vi "PID control-backup.vi"() -> ()   [LabVIEW 2017]
uses:
  <vilib>/Simulation/Scripting/Companion Diagram/SimConfigNode/SimParams.ctl
  <vilib>/Simulation/Scripting/Companion Diagram/SimConfigNode/_simSolvers.ctl
  <vilib>/Simulation/Implementation/Shared/SIMSCR Execution Mode.ctl
  <vilib>/Simulation/Param Hierarchy/Typedefs/SIMPH Param Control Actions.ctl
  <vilib>/Simulation/Implementation/Shared/NILVSim_ParamChanged.vi
  <vilib>/Simulation/Implementation/Shared/NILVSIM_BeginStep.vi
  <vilib>/Simulation/Implementation/Shared/NILVSim_Manager.vi
  <vilib>/Utility/error.llb/Clear Errors.vi
  <vilib>/Simulation/Implementation/Shared/NILVSim_FinalizeModel.vi
  <vilib>/DAQmx/read.llb/DAQmx Read (Counter DBL 1Chan 1Samp).vi
  <vilib>/DAQmx/read.llb/DAQmx Read (Digital Bool 1Line 1Point).vi
  917b7e52-755f-4d44-bea8-9e7c9beac24e.vi
  a58f9967-76f1-4ebc-ad3d-26e75a3ca160.vi
  <vilib>/DAQmx/write.llb/DAQmx Write (Analog DBL 1Chan 1Samp).vi
  <vilib>/DAQmx/create/channels.llb/DAQmx Create Channel (AO-Voltage-Basic).vi
  <vilib>/DAQmx/create/channels.llb/DAQmx Create Channel (DI-Digital Input).vi
  <vilib>/DAQmx/create/channels.llb/DAQmx Create Channel (CI-Count Edges).vi
  <vilib>/Simulation/Implementation/Shared/SIM Unbundle Sim Info.vi
  <vilib>/Simulation/Implementation/Shared/NILVSim_Initialize.vi
  <vilib>/Simulation/Utility/Implementation/NILVSim Get Time and IsAcceptedStep.vi
  <vilib>/Simulation/Implementation/Shared/SIMSH Read Queue.vi
  <vilib>/Simulation/Implementation/Shared/NILVSim_GetModelError.vi
  <vilib>/Simulation/Implementation/Shared/SIM Bundle Sim Info.vi
  <vilib>/DAQmx/miscellaneous.llb/DAQmx Fill In Error Info.vi
  <vilib>/Simulation/Implementation/XNodeFramework/SimXNode/SimX.xnode
  <vilib>/Simulation/Model Libraries/PID/SIM PID (Parallel).vi
  <vilib>/Simulation/Model Libraries/PID/SIM PID.vi
  <vilib>/Simulation/Scripting/Companion Diagram/SimConfigNode/SimDog.xnode
  <vilib>/Simulation/Model Libraries/PID/SIM PID (Academic).vi
  <vilib>/Simulation/Implementation/Shared/NI_SIM_Implementation.lvlib
panel:
  out "down":bool
  out "right":bool
  out "x entered":dbl
  out "y enetred":dbl
  out "Numeric 2":i32
  out "greater -1 x":bool
  out "less 1 x":bool
  out "d":bool
  out "c":bool
  out "b":bool
  out "direction selected":dbl
  out "circle reset":bool
  in  "part circle":T1(ring)=enum."a"
  in  "Raduis":dbl
  out "at 2f":bool
  out "Step 2J":bool
  out "Step 2H":bool
  out "Shape drawing steps":enum16{"corner", "1st switch", "reverse"}(ring)
  out "Step 2D":bool
  out "Step 2C":bool
  out "c":bool
  in  "height":dbl
  in  "length":dbl
  in  "part":T2(ring)=enum."a"
  out "Step 2A":bool
  out "Step 2B":bool
  in  "Has encoders been reset?":enum16{"don't reset", "reset"}(ring)
  out "x distance currently being travelled":dbl
  out "y distance currently being travelled":dbl
  out "error calced":dbl
  out "p1 dis 2":dbl
  out "p1 dis":dbl
  out "error y":dbl
  out "calc distance y":dbl
  out "calc distanc x":dbl
  out "error x":dbl
  out "reached y":bool
  out "reached x":bool
  out "Numeric":dbl
  in  "Draw rectangle":bool
  in  "Draw circle":bool
  out "In drawing mode":bool
  in  "Right-Down":bool
  in  "Left-Up":bool
  in  "Left-Down":bool
  in  "Right-Up":bool
  in  "right":bool
  in  "left":bool
  in  "motor 2":dbl(slide)=1.5 scale=-10.0..10.0
  in  "down":bool
  in  "up":bool
  in  "Y Length":dbl=30.0
  in  "X Length":dbl=30.0
  in  "Motor 2 encoder":tag="Dev1/ctr1"
  out "Pulses M2":dbl format="%.2f"
  in  "Motor 1 encoder":tag="Dev1/ctr0"
  out "Pulses M1":dbl format="%.2f"
  out "Right":bool
  out "Bottom":bool
  out "Left":bool
  out "Top":bool
  in  "Switch 4/Line 3":tag="Dev1/port0/line3"
  in  "Switch 3/Line 2":tag="Dev1/port0/line2"
  in  "Switch 2/Line 1":tag="Dev1/port0/line1"
  in  "Switch 1/Line 0":tag="Dev1/port0/line0"
  in  "Motor stop":bool
  in  "Motor 1":tag="Dev1/ao0"
  in  "max Voltage":dbl=10.0
  in  "Min Voltage":dbl=-10.0
  in  "Motor 2":tag="Dev1/ao1"
  in  "motor 1":dbl(slide)=1.5 scale=-10.0..10.0
  in  "stop":bool
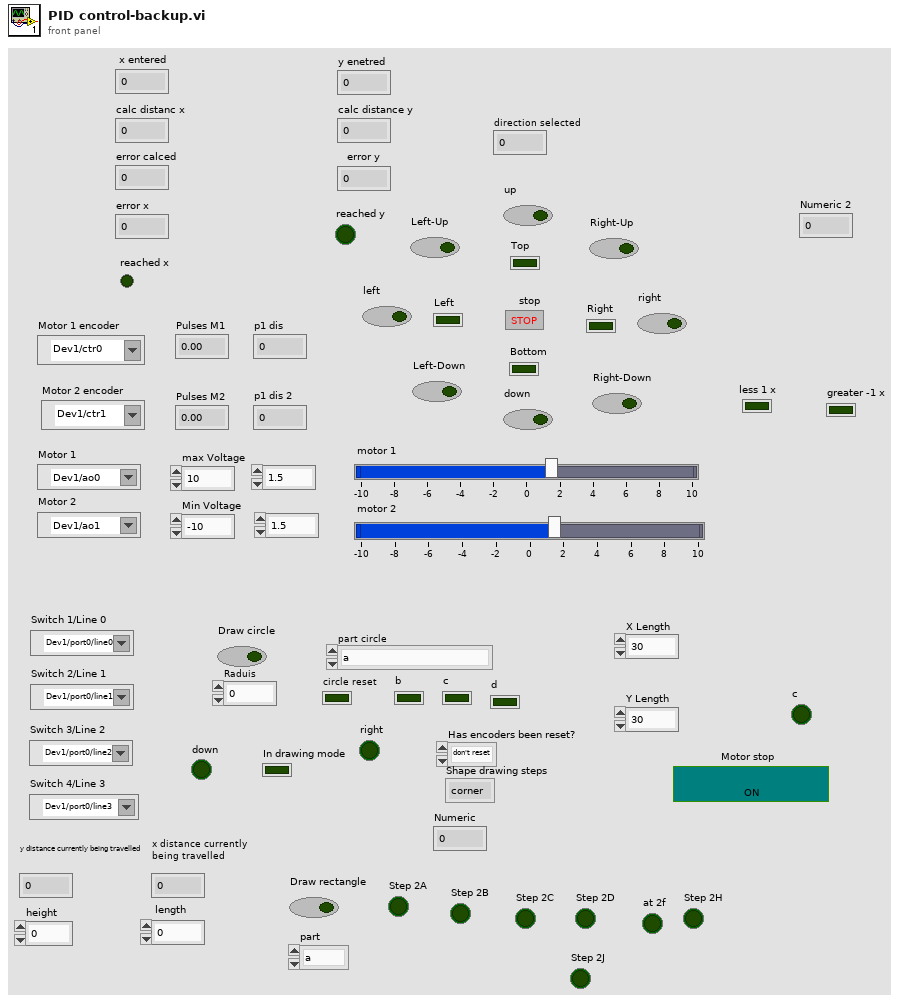
[diagram p1: front panel]
types:
  T1 = enum16{"d", "c", "b", "going right", "going down", "a"}
  T2 = enum16{"nothing", "j", "i", "h", "g", "f", "e", "d", "c", "b", "a"}
  T3 = enum16{"Simulate to Completion", "Single Time-Step Simulation (Fixed Step Only)"}
  T4 = typedef "SIMSCR Execution Mode.ctl" = enum16{"Simulate to Completion", "Single Time-Step Simulation (Fixed Step Only)"}
  T5 = typedef "SIMPH Param Control Actions.ctl" = enum16{"get params", "set params"}
  T6 = cluster{"SIMSH Sim Time":dbl, "SIM PID Derivative Gain.vi":cluster{"output":dbl}, "SIM PID Derivative Gain.vi - SIMSH":cluster{"SIMSH Sim Time":dbl, "t 3":dbl, "Select 2":cluster{"s? t:f":dbl}, "Equal?":cluster{"x = y?":bool}, "Or":cluster{"x .or. y?":bool}, "Equal To 0?":cluster{"x = 0?":bool}}, "High Frequency [s] (Tf)":dbl, "Gain":cluster{"output":dbl}, "Summation":cluster{"Result":dbl}, "Integral Gain - series.vi":cluster{"output":dbl}, "Integral Gain - series.vi - SIMSH":cluster{"SIMSH Sim Time":dbl, "Select 2":cluster{"s? t:f":dbl}, "integral in gain?":bool, "Integrator":cluster{"output y(t)":dbl}, "Gain 2":cluster{"output":dbl}, "Select":cluster{"s? t:f":dbl}, "Equal To 0?":cluster{"x = 0?":bool}, "Reciprocal":cluster{"1/x":dbl}}}
  T7 = typedef "SimParams.ctl" = cluster{"Initial Time (s)":dbl, "Final Time (s)":dbl, "Step Size (s)":dbl, "ODE Solver":T8, "Minimum Step Size (s)":dbl, "Maximum Step Size (s)":dbl, "Relative Tolerance":dbl, "Absolute Tolerance":dbl, "Software Timing":bool, "Initial Step Size (s)":dbl, "Automatic Fixed Step Size?":bool, "Automatic Discrete Step Size?":bool, "Discrete Step Size (s)":dbl, "Calculate using Time Step":bool, "Solver Wired?":bool, "Prev.Frm.Expected End":u64, "Prev.Frm.Actual End":u64, "Prev.Frm.Finished Late?":bool, "Prev.Iter.Expected End":u64, "Prev.Iter.Actual End":u64, "Prev.Iter.Finished Late?":bool, "Expected Iteration Start":u64, "Actual Iteration Start":u64, "Expected Frame Start":u64, "Actual Frame Start":u64, "Source Name":string, "Name":string, "Period":i64, "Deadline":i64, "Offset":i64, "Start":i64, "Priority":i32, "Timeout":i32, "Processor":i32, "Mode":enum32{"No Change", "Process missed periods, maintain original phase", "Discard missed periods, maintain original phase", "Process missed periods, ignore original phase", "Discard missed periods, ignore original phase"}, "Wakeup reason":enum32{"Normal", "Aborted", "Asynchronous wakeup", "Timing source error", "Timed loop error", "Timeout"}, "Error":errorcluster, "Source Type":string, "Secondary Source Type":string, "Global End Time":u64, "Global Start Time":u64, "Full Solver Reset":bool, "Execution Mode":T4, "Nan/Inf Check":bool, "Custom Solver Library":string, "Solver Is Variable":bool, "custom solver name":string, "Signal Collection Decimation":u32}
  T8 = typedef "_simSolvers.ctl" = enum16{"Runge-Kutta 1 (Euler)", "Runge-Kutta 2", "Runge-Kutta 3", "Runge-Kutta 4", "Runge-Kutta 23 (variable)", "Runge-Kutta 45 (variable)", "BDF (variable)", "Adams-Moulton (variable)", "Rosenbrock (variable)", "Discrete States Only", "SDIRK 4 (variable)", "Radau 5 (variable)", "Radau 9 (variable)", "Radau 13 (variable)", "Radau [Variable Order] (variable)", "Gear's Method (variable)", "Linearizer", "State Query", "Trim Eval", "Custom Solver"}
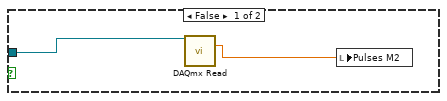
[diagram p2: hidden frame]
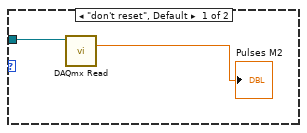
[diagram p3: hidden frame]
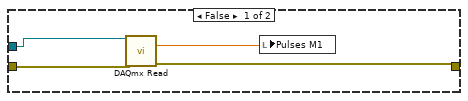
[diagram p4: hidden frame]
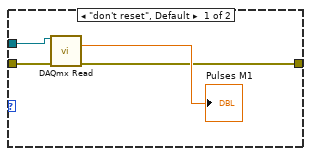
[diagram p5: hidden frame]
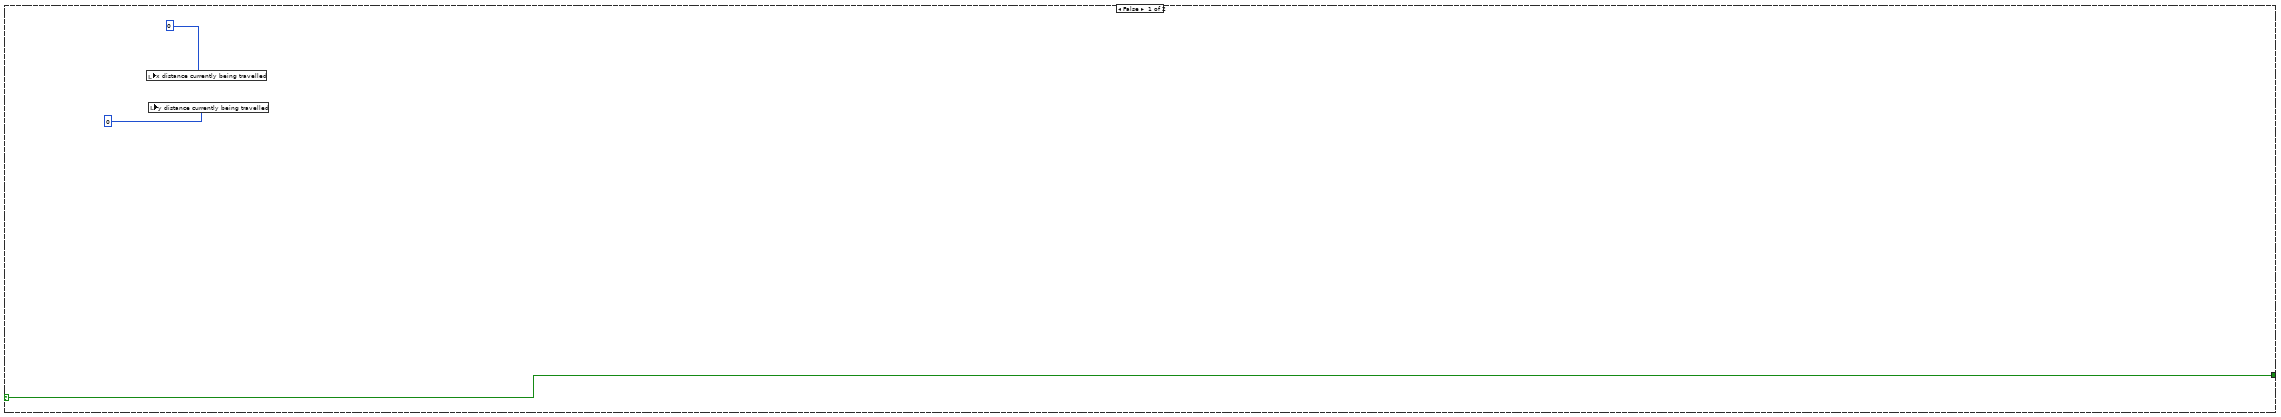
[diagram p6: hidden frame]
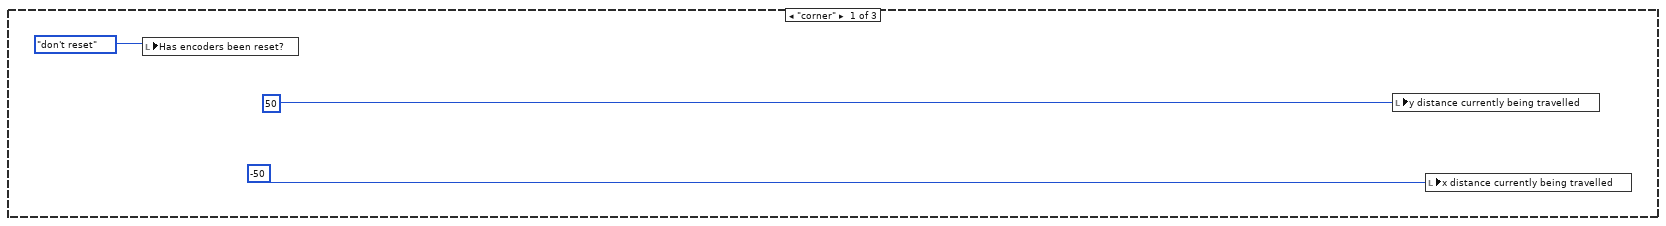
[diagram p7: hidden frame]
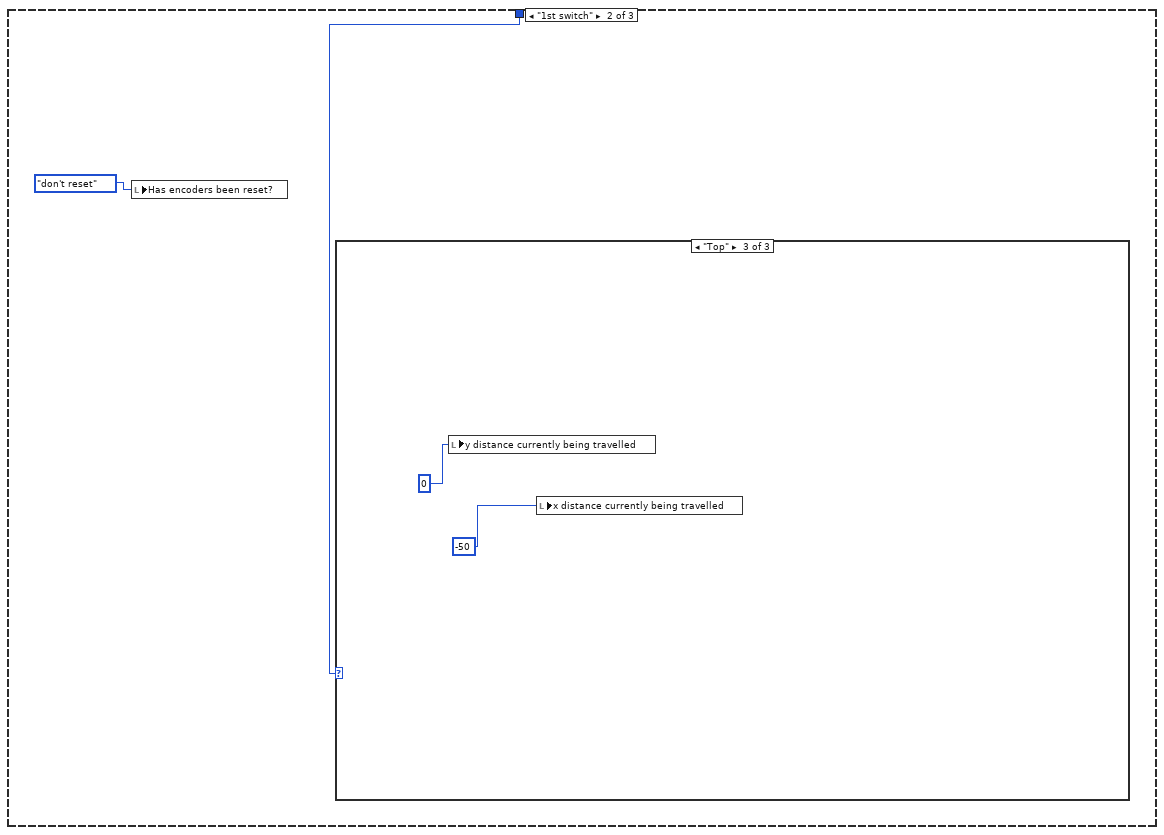
[diagram p8: hidden frame]
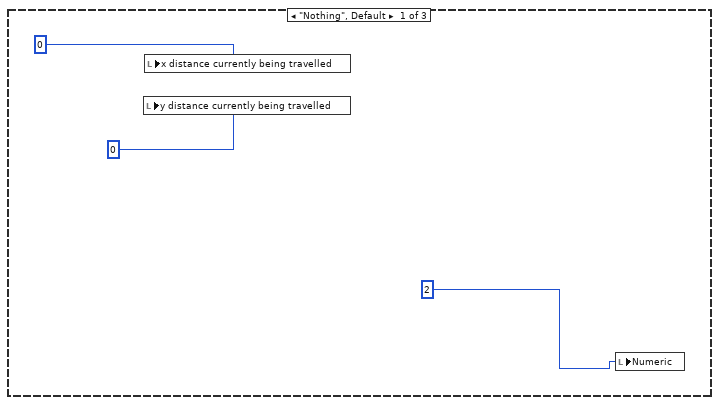
[diagram p9: hidden frame]
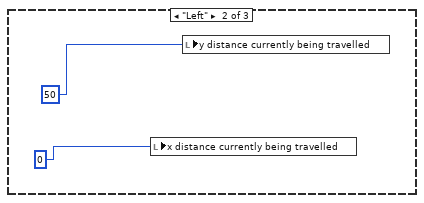
[diagram p10: hidden frame]
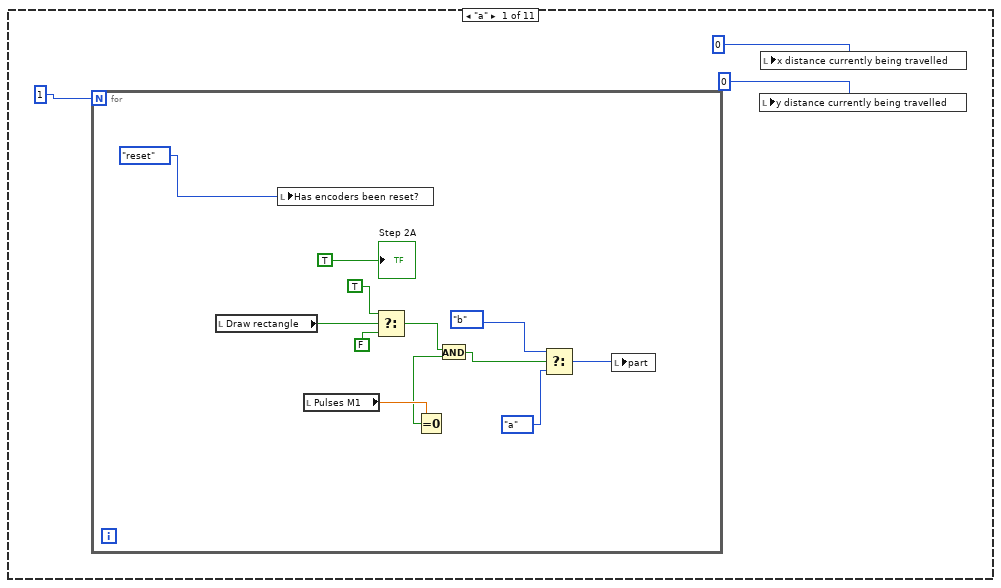
[diagram p11: hidden frame]
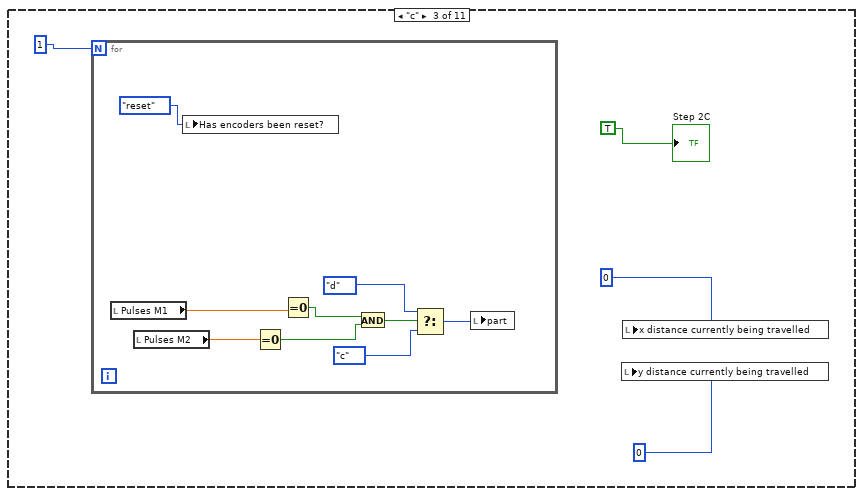
[diagram p12: hidden frame]
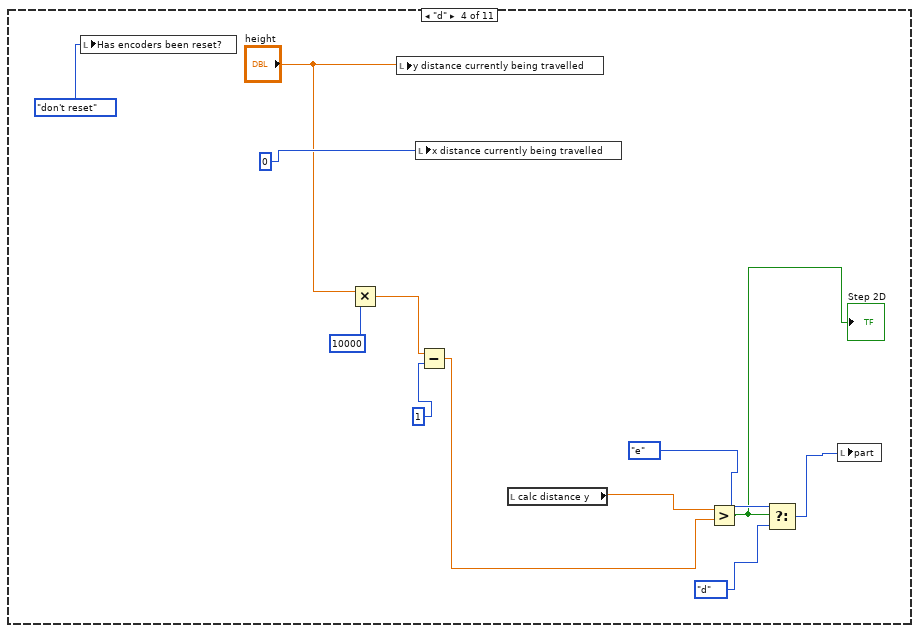
[diagram p13: hidden frame]
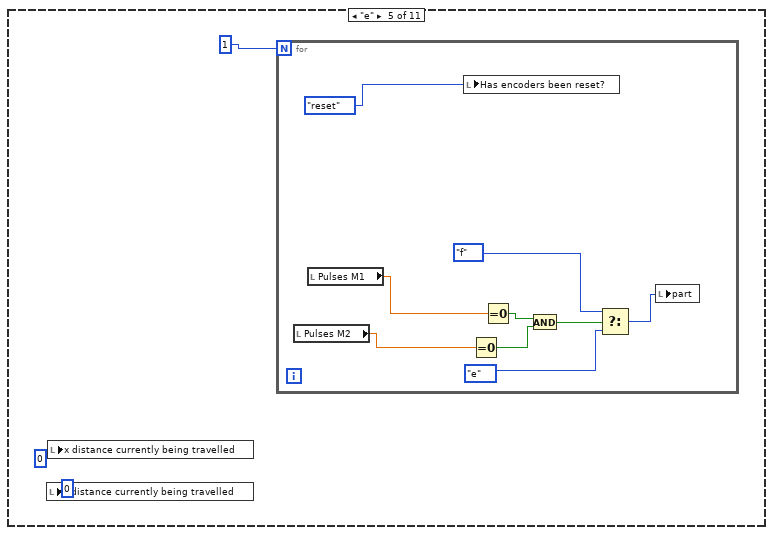
[diagram p14: hidden frame]
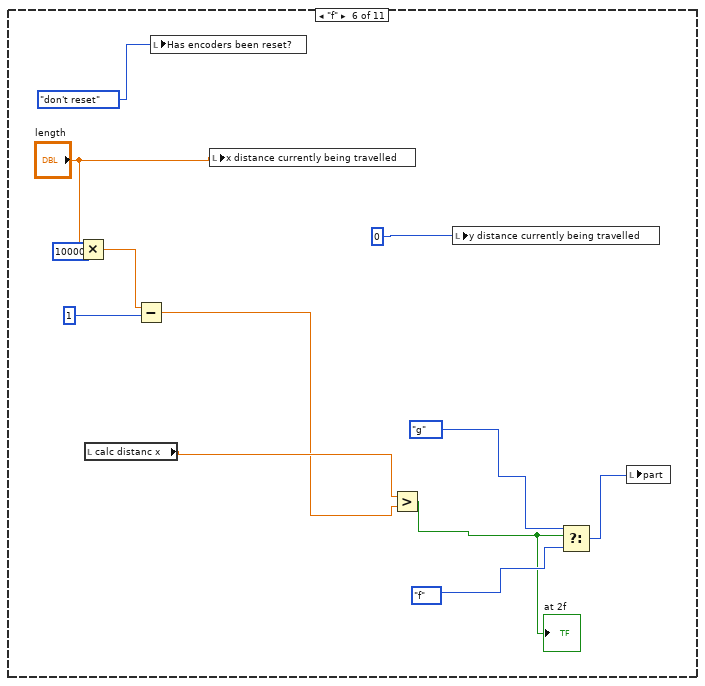
[diagram p15: hidden frame]
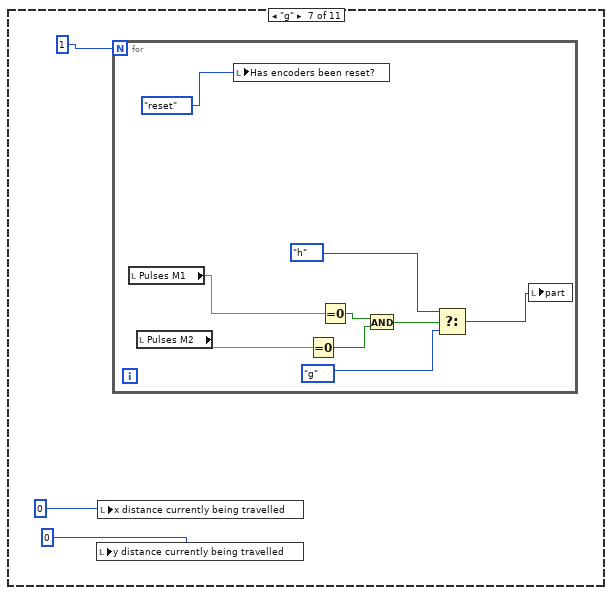
[diagram p16: hidden frame]
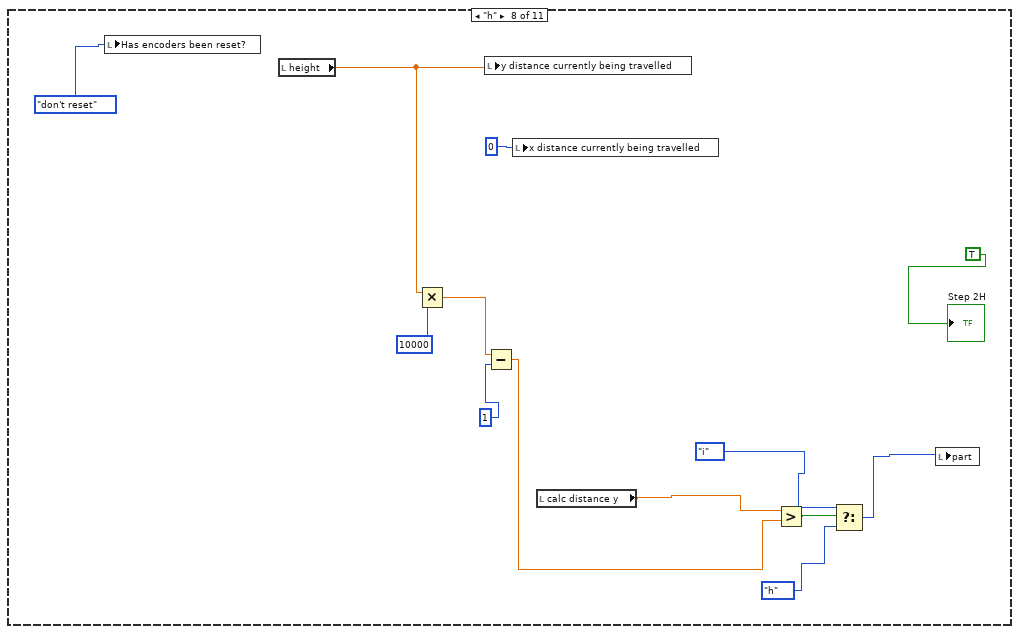
[diagram p17: hidden frame]
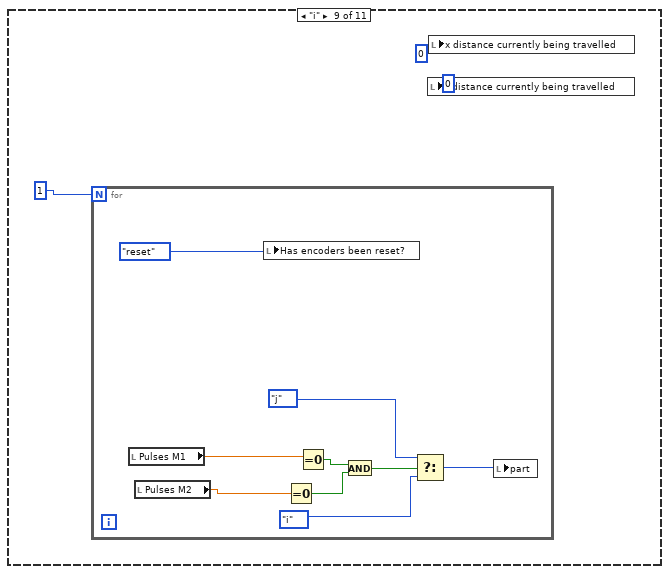
[diagram p18: hidden frame]
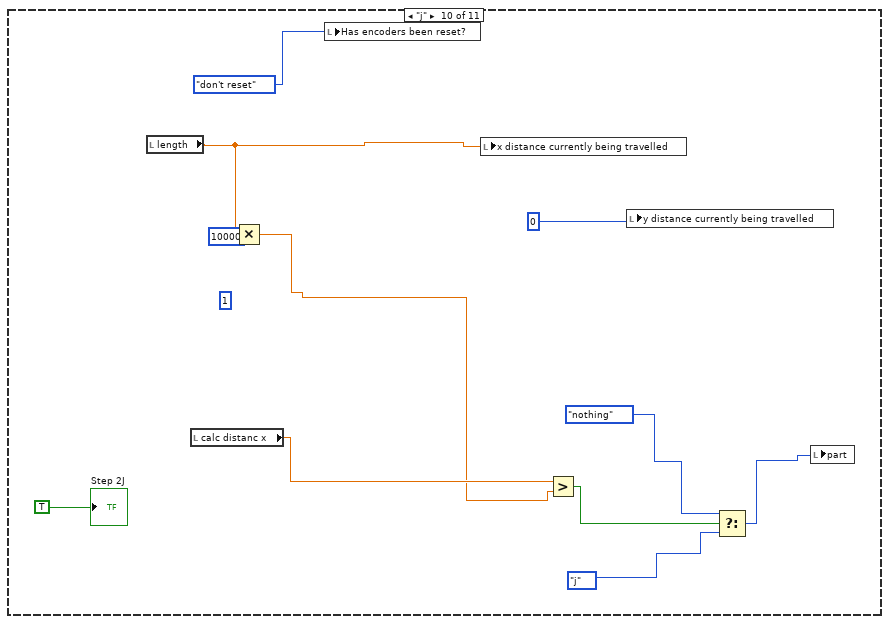
[diagram p19: hidden frame]
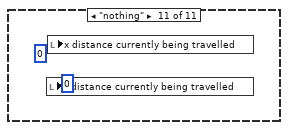
[diagram p20: hidden frame]
diagram:
  n1 = call-poly <vilib>:"DAQmx Create Virtual Channel.vi"("lines"="Switch 1/Line 0") -> ("task out"=w36:refnum<k21>, "error out"=w32:errorcluster)  [unwired: 13 in]
  n2 = call-poly <vilib>:"DAQmx Create Virtual Channel.vi"("lines"="Switch 2/Line 1") -> ("task out"=w35:refnum<k21>, "error out"=w31:errorcluster)  [unwired: 13 in]
  n3 = call-poly <vilib>:"DAQmx Create Virtual Channel.vi"("lines"="Switch 3/Line 2") -> ("task out"=w34:refnum<k21>, "error out"=w30:errorcluster)  [unwired: 13 in]
  n4 = call-poly <vilib>:"DAQmx Create Virtual Channel.vi"("lines"="Switch 4/Line 3") -> ("task out"=w33:refnum<k21>, "error out"=w29:errorcluster)  [unwired: 13 in]
  n5 = call <vilib>:"DAQmx Start Task.vi"("task/channels in"=w36, "error in"=w32) -> ("task out"=w28:refnum<k21>, "error out"=w26:errorcluster)  [unwired: 12 in]
  n6 = call <vilib>:"DAQmx Start Task.vi"("task/channels in"=w35, "error in"=w31) -> ("task out"=w24:refnum<k21>, "error out"=w21:errorcluster)  [unwired: 12 in]
  n7 = call <vilib>:"DAQmx Start Task.vi"("task/channels in"=w34, "error in"=w30) -> ("task out"=w23:refnum<k21>, "error out"=w20:errorcluster)  [unwired: 12 in]
  n8 = call <vilib>:"DAQmx Start Task.vi"("task/channels in"=w33, "error in"=w29) -> ("task out"=w22:refnum<k21>, "error out"=w19:errorcluster)  [unwired: 12 in]
  n9 = call-poly <vilib>:"DAQmx Create Virtual Channel.vi"("maximum value"="max Voltage", "minimum value"="Min Voltage", "physical channels"="Motor 1") -> ("task out"=w46:refnum<k21>, "error out"=w42:errorcluster)  [unwired: 11 in]
  n10 = call-poly <vilib>:"DAQmx Create Virtual Channel.vi"("counter"="Motor 2 encoder") -> ("task out"=w6:refnum<k21>)  [unwired: 13 in, 1 out]
  n11 = call-poly <vilib>:"DAQmx Create Virtual Channel.vi"("maximum value"="max Voltage", "minimum value"="Min Voltage", "physical channels"="Motor 2") -> ("task out"=w49:refnum<k21>, "error out"=w41:errorcluster)  [unwired: 11 in]
  n12 = call-poly <vilib>:"DAQmx Create Virtual Channel.vi"("counter"="Motor 1 encoder") -> ("task out"=w7:refnum<k21>, "error out"=w2:errorcluster)  [unwired: 13 in]
  n13 = call <vilib>:"DAQmx Start Task.vi"("task/channels in"=w6) -> ("task out"=w1:refnum<k21>)  [unwired: 13 in, 1 out]
  n14 = call <vilib>:"DAQmx Start Task.vi"("task/channels in"=w7) -> ("task out"=w3:refnum<k21>)  [unwired: 13 in, 1 out]
  n15 = while {
    tunnel: w49 -> [w239]
    tunnel: [w236] -> w48
    tunnel: w46 -> [w233]
    tunnel: [w232] -> w45
    tunnel: w42 -> [w230]
    tunnel: w41 -> [w229]
    tunnel: w28 -> [w223]
    tunnel: [w222] -> w27
    tunnel: w26 -> [w221]
    tunnel: [w220] -> w25
    tunnel: w24 -> [w219]
    tunnel: w23 -> [w218]
    tunnel: w22 -> [w217]
    tunnel: w21 -> [w216]
    tunnel: w20 -> [w215]
    tunnel: w19 -> [w214]
    tunnel: [w213] -> w18
    tunnel: [w212] -> w17
    tunnel: [w211] -> w16
    tunnel: [w210] -> w15
    tunnel: [w209] -> w14
    tunnel: [w208] -> w13
    tunnel: [w131] -> w10
    tunnel: w3 -> [w133]
    tunnel: w2 -> [w132]
    tunnel: w1 -> [w129]
    stop <- "stop" stop-if-true
    n16 = Or(x="Draw circle", y="Draw rectangle") -> (x .or. y?=w152:bool)
    n17 = local read "error y"() -> (w99:dbl)
    n18 = local read "error y"() -> (w98:dbl)
    n19 = local read "error x"() -> (w100:dbl)
    n20 = local read "error y"() -> (w114:dbl)
    n21 = local read "error y"() -> (w111:dbl)
    n22 = local read "error x"() -> (w107:dbl)
    n23 = local read "error x"() -> (w106:dbl)
    n24 = local read "error y"() -> (w115:dbl)
    n25 = local read "error x"() -> (w116:dbl)
    n26 = Less Than 0?(x=w99) -> (x < 0?=w97:bool)
    n27 = Less Than 0?(x=w100) -> (x < 0?=w96:bool)
    n28 = Greater Than 0?(x=w98) -> (x > 0?=w95:bool)
    n29 = Less Than 0?(x=w111) -> (x < 0?=w109:bool)
    n30 = Equal To 0?(x=w116) -> (x = 0?=w110:bool)
    n31 = Greater Than 0?(x=w114) -> (x > 0?=w113:bool)
    n32 = local read "error y"() -> (w92:dbl)
    n33 = local read "error x"() -> (w91:dbl)
    n34 = Greater Than 0?(x=w107) -> (x > 0?=w105:bool)
    n35 = Equal To 0?(x=w115) -> (x = 0?=w104:bool)
    n36 = Less Than 0?(x=w106) -> (x < 0?=w103:bool)
    n37 = And(x=w97, y=w96) -> (x .and. y?=w93:bool)
    n38 = And(x=w96, y=w95) -> (x .and. y?=w94:bool)
    n39 = And(x=w113, y=w110) -> (x .and. y?=w112:bool)
    n40 = And(x=w110, y=w109) -> (x .and. y?=w108:bool)
    n41 = local read "error y"() -> (w87:dbl)
    n42 = And(x=w105, y=w104) -> (x .and. y?=w102:bool)
    n43 = And(x=w104, y=w103) -> (x .and. y?=w101:bool)
    n44 = Greater Than 0?(x=w92) -> (x > 0?=w90:bool)
    n45 = Greater Than 0?(x=w91) -> (x > 0?=w88:bool)
    n46 = Less Than 0?(x=w87) -> (x < 0?=w86:bool)
    n47 = And(x=w90, y=w88) -> (x .and. y?=w89:bool)
    n48 = And(x=w88, y=w86) -> (x .and. y?=w85:bool)
    n49 = Select(t=1, s=w112, f=0) -> (s? t:f=w192:i32)
    n50 = Select(t=10, s=w101, f=0) -> (s? t:f=w190:i32)
    n51 = Select(t=2, s=w108, f=0) -> (s? t:f=w191:i32)
    n52 = Select(t=100, s=w89, f=0) -> (s? t:f=w188:i32)
    n53 = Select(t=200, s=w93, f=0) -> (s? t:f=w187:i32)
    n54 = Select(t=20, s=w102, f=0) -> (s? t:f=w189:i32)
    n55 = Select(t=1000, s=w94, f=0) -> (s? t:f=w186:i32)
    n56 = Select(t=2000, s=w85, f=0) -> (s? t:f=w172:i32)
    n57 = Add(x=w192, y=w191) -> (x+y=w185:i32)
    n58 = Add(x=w190, y=w189) -> (x+y=w184:i32)
    n59 = Add(x=w188, y=w187) -> (x+y=w183:i32)
    n60 = Add(x=w186, y=w172) -> (x+y=w171:i32)
    n61 = Add(x=w185, y=w184) -> (x+y=w182:i32)
    n62 = local read "y distance currently being travelled"() -> (w135:dbl)
    n63 = Add(x=w183, y=w171) -> (x+y=w170:i32)
    n64 = local read "Draw rectangle"() -> (w143:bool)
    n65 = local read "Draw circle"() -> (w144:bool)
    n66 = call-poly <vilib>:"DAQmx Read.vi"("task/channels in"=w223, "error in"=w221) -> ("task out"=w222:refnum<k21>, "data"=w154:bool, "error out"=w220:errorcluster)  [unwired: 11 in]
    "Top" <- w154
    n67 = call-poly <vilib>:"DAQmx Read.vi"("task/channels in"=w219, "error in"=w216) -> ("task out"=w213:refnum<k21>, "data"=w163:bool, "error out"=w210:errorcluster)  [unwired: 11 in]
    "Bottom" <- w163
    n68 = call-poly <vilib>:"DAQmx Read.vi"("task/channels in"=w218, "error in"=w215) -> ("task out"=w212:refnum<k21>, "data"=w162:bool, "error out"=w209:errorcluster)  [unwired: 11 in]
    "Right" <- w162
    n69 = call-poly <vilib>:"DAQmx Read.vi"("task/channels in"=w217, "error in"=w214) -> ("task out"=w211:refnum<k21>, "data"=w161:bool, "error out"=w208:errorcluster)  [unwired: 11 in]
    "Left" <- w161
    n70 = Add(x=w182, y=w170) -> (x+y=w84:i32)
    "direction selected" <- w84
    n71 = Or(x=w144, y=w143) -> (x .or. y?=w142:bool)
    n72 = Select(t=w135, s=w142, f="Y Length") -> (s? t:f=w140:dbl)
    n73 = Multiply(x=w140, y=10) -> (x*y=w54:dbl)
    "y enetred" <- w54
    n74 = local read "Pulses M1"() -> (w130:dbl)
    n75 = local read "Pulses M2"() -> (w145:dbl)
    n76 = Divide(x=w130, y=52.56) -> (x/y=→"p1 dis":dbl)
    n77 = feedback #1() -> (w58:dbl)  [unwired: 1 in]
    "calc distance y" <- w58
    n78 = formula code="if (Ylength==0)\nYerror=0;\n else  \nif(Ylength<0)\nYerror= Ylength+calculating_y_dis;\nelse\nYerror= Ylength-calculating_y_dis;\n\nif (calculating_y_dis>1000)\nstay=0;\nif (stay==0 )\nYerror=0;"("Ylength"=w54, "calculating_y_dis"=w58, "stay"=1) -> ("Yerror"=w118:dbl)
    n79 = Divide(x=w145, y=52.56) -> (x/y=→"p1 dis 2":dbl)
    n80 = formula code="X=((PulseM1/52.56)+(PulseM2/52.56))/2.0;\nY=((PulseM1/52.56)+(PulseM2/52.56))/2.0;"("PulseM1"=w130, "PulseM2"=w145) -> ("X"=w63:dbl, "Y"=w67:dbl)
    n81 = local read "x distance currently being travelled"() -> (w134:dbl)
    n82 = local read "Draw rectangle"() -> (w137:bool)
    n83 = Multiply(x=1000, y=w67) -> (x*y=w70:dbl)
    n84 = local read "Draw circle"() -> (w136:bool)
    n85 = xnode "PID"("Error"=w118) -> ("Output"=w69:dbl)  [unwired: 2 in, 11 out]
    n86 = Or(x=w137, y=w136) -> (x .or. y?=w125:bool)
    n87 = Select(t=w134, s=w125, f="X Length") -> (s? t:f=w138:dbl)
    n88 = Multiply(x=w138, y=10) -> (x*y=w53:dbl)
    "x entered" <- w53
    n89 = Multiply(x=1000, y=w63) -> (x*y=w64:dbl)
    n90 = Greater?(x=1, y=w69) -> (0:w82:bool)
    n91 = Less?(x=-1, y=w69) -> (x < y?=w80:bool)
    n92 = case shown="2000" w84 {
      tunnel: "motor 1" -> [w996 w999 w1002 w1009 w1013 w1017 w1023 w1029 w1035 w1040 w1047]
      tunnel: "motor 2" -> [w993 w1001 w1004 w1007 w1012 w1015 w1021 w1027 w1033 w1041 w1046]
      tunnel: [w992 w1001 w1003 w1006 w1012 w1014 w1020 w1026 w1032 w1038 w1045] -> w51
      tunnel: [w995 w998 w1002 w1008 w1013 w1016 w1022 w1028 w1034 w1039 w1044] -> w52
      frame 0, Default {
        n93 = Multiply(x=0, y=w996) -> (x*y=w995:dbl)
        n94 = Multiply(x=0, y=w993) -> (x*y=w992:dbl)
      }
      frame 1 {
        n95 = Multiply(x=-1, y=w999) -> (x*y=w998:dbl)
      }
      frame 2 {
        n96 = Multiply(x=-1.003, y=w1004) -> (x*y=w1003:dbl)
      }
      frame 10 {
        n97 = Multiply(x=-1, y=w1009) -> (x*y=w1008:dbl)
        n98 = Multiply(x=-1.1, y=w1007) -> (x*y=w1006:dbl)
      }
      frame 20 {
      }
      frame 100 {
        n99 = Multiply(x=0, y=w1017) -> (x*y=w1016:dbl)
        n100 = Multiply(x=1, y=w1015) -> (x*y=w1014:dbl)
      }
      frame 200 {
        n101 = Multiply(x=0, y=w1023) -> (x*y=w1022:dbl)
        n102 = Multiply(x=-1, y=w1021) -> (x*y=w1020:dbl)
      }
      frame 1000 {
        n103 = Multiply(x=-1, y=w1029) -> (x*y=w1028:dbl)
        n104 = Multiply(x=0, y=w1027) -> (x*y=w1026:dbl)
      }
      frame 2000 {
        n105 = Multiply(x=1, y=w1035) -> (x*y=w1034:dbl)
        n106 = Multiply(x=0, y=w1033) -> (x*y=w1032:dbl)
      }
      frame 4000 {
        n107 = Multiply(x=-1, y=w1040) -> (x*y=w1039:dbl)
        n108 = Multiply(x=0, y=w1041) -> (x*y=w1038:dbl)
      }
      frame 8000 {
        n109 = Multiply(x=-1, y=w1047) -> (x*y=w1044:dbl)
        n110 = Multiply(x=0, y=w1046) -> (x*y=w1045:dbl)
      }
    }
    n111 = And(x=w82, y=w80) -> (x .and. y?=w68:bool)
    "reached y" <- w68
    n112 = Select(t=w70, s=w68, f=w67) -> (s? t:f=w66:dbl)
    n113 = feedback-in #1(w66) -> ()
    n114 = Multiply(x=0, y=w69) -> (x*y=w78:dbl)
    n115 = Select(t=w78, s=w68, f=w69) -> (s? t:f=→"error y":dbl)
    n116 = local read "Numeric"() -> (w122:dbl)
    n117 = Or(x=w163, y=w162) -> (x .or. y?=w206:bool)
    n118 = local read "Draw circle"() -> (w127:bool)
    n119 = local read "Draw rectangle"() -> (w126:bool)
    n120 = And(x=w161, y=w154) -> (x .and. y?=w123:bool)
    n121 = Exclusive Or(1:w154, 2:w161) -> (0:w168:bool)
    n122 = Select(t=1, s=w161, f=0) -> (s? t:f=w153:i32)
    n123 = Select(t=2, s=w154, f=w153) -> (s? t:f=w158:i32)
    n124 = Select(t=1, s=w168, f=w122) -> (s? t:f=w167:dbl)
    n125 = Select(t=2, s=w123, f=w167) -> (s? t:f=w165:dbl)
    n126 = feedback #2() -> (w61:bool)  [unwired: 1 in]
    "reached x" <- w61
    n127 = Select(t=w64, s=w61, f=w63) -> (s? t:f=w57:dbl)
    "calc distanc x" <- w57
    n128 = formula code="if (actual_xLength>1000)\nstay1=0;\nif (stay1==0)\nXerror=0;\nelse \nif(desired_xlength>0)\nXerror=desired_xlength-actual_xLength;\nelse\nXerror=desired_xlength+actual_xLength;"("actual_xLength"=w57, "desired_xlength"=w53, "stay1"=1) -> ("Xerror"=w117:dbl)
    "error calced" <- w117
    n129 = xnode "PID 2"("Error"=w117) -> ("Output"=w73:dbl)  [unwired: 2 in, 11 out]
    n130 = Greater?(x=1, y=w73) -> (0:w59:bool)
    "greater -1 x" <- w59
    n131 = Less?(x=-1, y=w73) -> (x < y?=w60:bool)
    "less 1 x" <- w60
    n132 = And(x=w59, y=w60) -> (x .and. y?=w62:bool)
    n133 = Multiply(x=0, y=w73) -> (x*y=w75:dbl)
    n134 = feedback-in #2(w62) -> ()
    n135 = Or(x=w127, y=w126) -> (x .or. y?=w128:bool)
    n136 = Select(t=w75, s=w61, f=w73) -> (s? t:f=→"error x":dbl)
    n137 = call "Number To Enum.vim"("number"=w158, "enum type"=enum16{"Nothing", "Left", "Top"}."Left") -> ("number as enum"=w155:enum16{"Nothing", "Left", "Top"})
    n138 = case shown="True" w152 {
      selector: w152 -> [w766 w774]
      tunnel: [w766 w774] -> w169
      tunnel: w155 -> [_ w767]
      frame False {
        n139 = local write "x distance currently being travelled"(0) -> ()
        n140 = local write "y distance currently being travelled"(0) -> ()
      }
      frame True {
        n141 = local read "Numeric"() -> (w772:dbl)
        n142 = local read "Shape drawing steps"() -> (w769:enum16{"corner", "1st switch", "reverse"})
        n143 = Equal?(x=w772, y=2) -> (x = y?=w771:bool)
        n144 = Select(t=enum16{"corner", "1st switch", "reverse"}."reverse", s=w771, f=w769) -> (s? t:f=w768:enum16{"corner", "1st switch", "reverse"})
        n145 = case shown="\"reverse\"" w768 {
          tunnel: w767 -> [_ w778 _]
          frame "corner" {
            n146 = local write "Has encoders been reset?"(enum16{"don't reset", "reset"}."don't reset") -> ()
            n147 = local write "y distance currently being travelled"(50) -> ()
            n148 = local write "x distance currently being travelled"(-50) -> ()
          }
          frame "1st switch" {
            n149 = local write "Has encoders been reset?"(enum16{"don't reset", "reset"}."don't reset") -> ()
            n150 = case shown="\"Top\"" w778 {
              frame "Nothing", Default {
                n151 = local write "y distance currently being travelled"(0) -> ()
                n152 = local write "x distance currently being travelled"(0) -> ()
                n153 = local write "Numeric"(2) -> ()
              }
              frame "Left" {
                n154 = local write "x distance currently being travelled"(0) -> ()
                n155 = local write "y distance currently being travelled"(50) -> ()
              }
              frame "Top" {
                n156 = local write "y distance currently being travelled"(0) -> ()
                n157 = local write "x distance currently being travelled"(-50) -> ()
              }
            }
          }
          frame "reverse" {
            n158 = local read "Draw circle"() -> (w787:bool)
            n159 = case shown="False" w787 {
              tunnel: "part" -> [w790 _]
              frame False {
                n160 = case shown="\"b\"" w790 {
                  frame "a" {
                    n161 = for {
                      N: 1 -> [_]
                      n162 = local read "Draw rectangle"() -> (w794:bool)
                      n163 = local write "Has encoders been reset?"(enum16{"don't reset", "reset"}."reset") -> ()
                      n164 = local read "Pulses M1"() -> (w803:dbl)
                      n165 = Select(t=TRUE, s=w794, f=FALSE) -> (s? t:f=w797:bool)
                      n166 = Equal To 0?(x=w803) -> (x = 0?=w796:bool)
                      n167 = And(x=w797, y=w796) -> (x .and. y?=w795:bool)
                      n168 = Select(t=T2."b", s=w795, f=T2."a") -> (s? t:f=w802:T2)
                      n169 = local write "part"(w802) -> ()
                      "Step 2A" <- TRUE
                    }
                    n170 = local write "y distance currently being travelled"(0) -> ()
                    n171 = local write "x distance currently being travelled"(0) -> ()
                  }
                  frame "b" {
                    n172 = local read "calc distance y"() -> (w806:dbl)
                    n173 = local read "calc distanc x"() -> (w807:dbl)
                    n174 = local write "Has encoders been reset?"(enum16{"don't reset", "reset"}."don't reset") -> ()
                    n175 = Greater?(x=w806, y=9000) -> (0:w812:bool)
                    n176 = Greater?(x=w807, y=29000) -> (0:w811:bool)
                    n177 = And(x=w811, y=w812) -> (x .and. y?=w810:bool)
                    "c" <- w810
                    n178 = Select(t=T2."c", s=w810, f=T2."b") -> (s? t:f=w815:T2)
                    n179 = local write "part"(w815) -> ()
                    "x distance currently being travelled" <- 3
                    "y distance currently being travelled" <- 1
                    "Step 2B" <- TRUE
                  }
                  frame "c" {
                    n180 = for {
                      N: 1 -> [_]
                      n181 = local read "Pulses M1"() -> (w831:dbl)
                      n182 = local read "Pulses M2"() -> (w827:dbl)
                      n183 = local write "Has encoders been reset?"(enum16{"don't reset", "reset"}."reset") -> ()
                      n184 = Equal To 0?(x=w827) -> (x = 0?=w825:bool)
                      n185 = Equal To 0?(x=w831) -> (x = 0?=w826:bool)
                      n186 = And(x=w826, y=w825) -> (x .and. y?=w824:bool)
                      n187 = Select(t=T2."d", s=w824, f=T2."c") -> (s? t:f=w830:T2)
                      n188 = local write "part"(w830) -> ()
                    }
                    n189 = local write "y distance currently being travelled"(0) -> ()
                    n190 = local write "x distance currently being travelled"(0) -> ()
                    "Step 2C" <- TRUE
                  }
                  frame "d" {
                    n191 = local write "Has encoders been reset?"(enum16{"don't reset", "reset"}."don't reset") -> ()
                    n192 = Multiply(x="height", y=10000) -> (x*y=w840:dbl)
                    n193 = local write "y distance currently being travelled"("height") -> ()
                    n194 = local write "x distance currently being travelled"(0) -> ()
                    n195 = Subtract(x=w840, y=1) -> (x-y=w837:dbl)
                    n196 = local read "calc distance y"() -> (w842:dbl)
                    n197 = Greater?(x=w842, y=w837) -> (0:w833:bool)
                    "Step 2D" <- w833
                    n198 = Select(t=T2."e", s=w833, f=T2."d") -> (s? t:f=w843:T2)
                    n199 = local write "part"(w843) -> ()
                  }
                  frame "e" {
                    n200 = local write "y distance currently being travelled"(0) -> ()
                    n201 = local write "x distance currently being travelled"(0) -> ()
                    n202 = for {
                      N: 1 -> [_]
                      n203 = local read "Pulses M2"() -> (w849:dbl)
                      n204 = local read "Pulses M1"() -> (w850:dbl)
                      n205 = local write "Has encoders been reset?"(enum16{"don't reset", "reset"}."reset") -> ()
                      n206 = Equal To 0?(x=w849) -> (x = 0?=w855:bool)
                      n207 = Equal To 0?(x=w850) -> (x = 0?=w856:bool)
                      n208 = And(x=w856, y=w855) -> (x .and. y?=w854:bool)
                      n209 = Select(t=T2."f", s=w854, f=T2."e") -> (s? t:f=w848:T2)
                      n210 = local write "part"(w848) -> ()
                    }
                  }
                  frame "f" {
                    n211 = Multiply(x="length", y=10000) -> (x*y=w863:dbl)
                    n212 = local read "calc distanc x"() -> (w866:dbl)
                    n213 = Subtract(x=w863, y=1) -> (x-y=w860:dbl)
                    n214 = local write "Has encoders been reset?"(enum16{"don't reset", "reset"}."don't reset") -> ()
                    n215 = local write "x distance currently being travelled"("length") -> ()
                    n216 = Greater?(x=w866, y=w860) -> (0:w857:bool)
                    "at 2f" <- w857
                    n217 = local write "y distance currently being travelled"(0) -> ()
                    n218 = Select(t=T2."g", s=w857, f=T2."f") -> (s? t:f=w865:T2)
                    n219 = local write "part"(w865) -> ()
                  }
                  frame "g" {
                    n220 = local write "y distance currently being travelled"(0) -> ()
                    n221 = local write "x distance currently being travelled"(0) -> ()
                    n222 = for {
                      N: 1 -> [_]
                      n223 = local read "Pulses M1"() -> (w873:dbl)
                      n224 = local read "Pulses M2"() -> (w872:dbl)
                      n225 = local write "Has encoders been reset?"(enum16{"don't reset", "reset"}."reset") -> ()
                      n226 = Equal To 0?(x=w872) -> (x = 0?=w879:bool)
                      n227 = Equal To 0?(x=w873) -> (x = 0?=w880:bool)
                      n228 = And(x=w880, y=w879) -> (x .and. y?=w878:bool)
                      n229 = Select(t=T2."h", s=w878, f=T2."g") -> (s? t:f=w875:T2)
                      n230 = local write "part"(w875) -> ()
                    }
                  }
                  frame "h" {
                    n231 = local write "Has encoders been reset?"(enum16{"don't reset", "reset"}."don't reset") -> ()
                    n232 = local read "height"() -> (w884:dbl)
                    n233 = Multiply(x=w884, y=10000) -> (x*y=w892:dbl)
                    n234 = local write "y distance currently being travelled"(w884) -> ()
                    n235 = Subtract(x=w892, y=1) -> (x-y=w889:dbl)
                    n236 = local write "x distance currently being travelled"(0) -> ()
                    n237 = local read "calc distance y"() -> (w882:dbl)
                    n238 = Greater?(x=w882, y=w889) -> (0:w893:bool)
                    n239 = Select(t=T2."i", s=w893, f=T2."h") -> (s? t:f=w885:T2)
                    n240 = local write "part"(w885) -> ()
                    "Step 2H" <- TRUE
                  }
                  frame "i" {
                    n241 = for {
                      N: 1 -> [_]
                      n242 = local read "Pulses M1"() -> (w899:dbl)
                      n243 = local read "Pulses M2"() -> (w898:dbl)
                      n244 = local write "Has encoders been reset?"(enum16{"don't reset", "reset"}."reset") -> ()
                      n245 = Equal To 0?(x=w898) -> (x = 0?=w904:bool)
                      n246 = Equal To 0?(x=w899) -> (x = 0?=w905:bool)
                      n247 = And(x=w905, y=w904) -> (x .and. y?=w903:bool)
                      n248 = Select(t=T2."j", s=w903, f=T2."i") -> (s? t:f=w897:T2)
                      n249 = local write "part"(w897) -> ()
                    }
                    n250 = local write "y distance currently being travelled"(0) -> ()
                    n251 = local write "x distance currently being travelled"(0) -> ()
                  }
                  frame "j" {
                    (unwired) 1
                    n252 = local read "length"() -> (w909:dbl)
                    n253 = local read "calc distanc x"() -> (w911:dbl)
                    n254 = Multiply(x=w909, y=10000) -> (x*y=w906:dbl)
                    n255 = local write "Has encoders been reset?"(enum16{"don't reset", "reset"}."don't reset") -> ()
                    n256 = local write "x distance currently being travelled"(w909) -> ()
                    n257 = Greater?(x=w911, y=w906) -> (0:w914:bool)
                    n258 = local write "y distance currently being travelled"(0) -> ()
                    n259 = Select(t=T2."nothing", s=w914, f=T2."j") -> (s? t:f=w910:T2)
                    n260 = local write "part"(w910) -> ()
                    "Step 2J" <- TRUE
                  }
                  frame "nothing" {
                    n261 = local write "y distance currently being travelled"(0) -> ()
                    n262 = local write "x distance currently being travelled"(0) -> ()
                  }
                }
              }
              frame True {
                n263 = case shown="\"b\"" "part circle" {
                  frame "a" {
                    n264 = for {
                      N: 1 -> [_]
                      n265 = local read "Pulses M1"() -> (w926:dbl)
                      n266 = local read "Pulses M2"() -> (w925:dbl)
                      n267 = Equal To 0?(x=w926) -> (x = 0?=w928:bool)
                      n268 = Equal To 0?(x=w925) -> (x = 0?=w929:bool)
                      n269 = And(x=w928, y=w929) -> (x .and. y?=w930:bool)
                      n270 = local write "Has encoders been reset?"(enum16{"don't reset", "reset"}."reset") -> ()
                      n271 = Select(t=T1."going down", s=w930, f=T1."a") -> (s? t:f=w923:T1)
                      n272 = local write "part circle"(w923) -> ()
                      "circle reset" <- TRUE
                    }
                  }
                  frame "going down" {
                    n273 = local read "calc distance y"() -> (w938:dbl)
                    n274 = Greater?(x=w938, y=38000) -> (0:w934:bool)
                    n275 = local write "Has encoders been reset?"(enum16{"don't reset", "reset"}."don't reset") -> ()
                    n276 = Select(t=T1."going right", s=w934, f=T1."going right") -> (s? t:f=w933:T1)
                    n277 = local write "y distance currently being travelled"(-2) -> ()
                    n278 = local write "part circle"(w933) -> ()
                    "down" <- TRUE
                  }
                  frame "going right" {
                    n279 = local write "Has encoders been reset?"(enum16{"don't reset", "reset"}."reset") -> ()
                    n280 = local write "part circle"(T1."b") -> ()
                    "right" <- TRUE
                  }
                  frame "b" {
                    n281 = local read "Raduis"() -> (w959:dbl)
                    n282 = local read "calc distanc x"() -> (w956:dbl)
                    n283 = local read "calc distance y"() -> (w955:dbl)
                    n284 = Multiply(x=w959, y=10) -> (x*y=w958:dbl)
                    n285 = Subtract(x=w958, y=1) -> (x-y=w947:dbl)
                    n286 = local read "Raduis"() -> (w950:dbl)
                    n287 = Multiply(x=-1, y=w950) -> (x*y=w949:dbl)
                    n288 = Greater?(x=w956, y=w947) -> (0:w954:bool)
                    n289 = local write "y distance currently being travelled"(w949) -> ()
                    n290 = Multiply(x=-1, y=w947) -> (x*y=w946:dbl)
                    n291 = Greater?(x=w955, y=w946) -> (0:w953:bool)
                    n292 = local write "x distance currently being travelled"(w950) -> ()
                    n293 = And(x=w954, y=w953) -> (x .and. y?=w952:bool)
                    "b" <- w952
                    n294 = local write "Has encoders been reset?"(enum16{"don't reset", "reset"}."don't reset") -> ()
                    n295 = Select(t=T1."c", s=w952, f=T1."b") -> (s? t:f=w943:T1)
                    n296 = local write "part circle"(w943) -> ()
                  }
                  frame "c" {
                    n297 = for {
                      N: 1 -> [_]
                      n298 = local read "Pulses M1"() -> (w969:dbl)
                      n299 = local read "Pulses M2"() -> (w968:dbl)
                      n300 = Equal To 0?(x=w969) -> (x = 0?=w970:bool)
                      n301 = Equal To 0?(x=w968) -> (x = 0?=w971:bool)
                      n302 = local write "Has encoders been reset?"(enum16{"don't reset", "reset"}."reset") -> ()
                      n303 = And(x=w970, y=w971) -> (x .and. y?=w965:bool)
                      "c" <- w965
                      n304 = Select(t=T1."d", s=w965, f=T1."c") -> (s? t:f=w966:T1)
                      n305 = local write "part circle"(w966) -> ()
                    }
                  }
                  frame "d" {
                    n306 = while {
                      i -> [w981]
                      stop <- w980 stop-if-true
                      n307 = for {
                        N: 50 -> [_]
                        tunnel: [w984] -> w974
                        i -> [w989]
                        n308 = Increment(x=w989) -> (x+1=w985:i32)
                        "Numeric 2" <- w985
                        n309 = Multiply(x=2, y=3.141592653589793) -> (x*y=w986:dbl)
                        n310 = Divide(x=w986, y=50) -> (x/y=w988:dbl)
                        n311 = Multiply(x=w988, y=w985) -> (x*y=w984:dbl)
                      }
                      n312 = Equal?(x=49, y=w981) -> (x = y?=w980:bool)
                      n313 = local write "Has encoders been reset?"(enum16{"don't reset", "reset"}."don't reset") -> ()
                      n314 = Cosine(x=w974) -> (cos(x)=w976:dbl)
                      n315 = Sine(x=w974) -> (sin(x)=w977:dbl)
                      n316 = Multiply(x=w977, y="Raduis") -> (x*y=w979:dbl)
                      n317 = Multiply(x=w976, y="Raduis") -> (x*y=w978:dbl)
                      n318 = local write "x distance currently being travelled"(w978) -> ()
                      n319 = local write "y distance currently being travelled"(w979) -> ()
                      "d" <- TRUE
                    }
                  }
                }
              }
            }
            "Numeric" <- 2
          }
        }
      }
    }
    "In drawing mode" <- w169
    n320 = And(x=w68, y=w61) -> (x .and. y?=w151:bool)
    n321 = Or(x=w206, y=w151) -> (x .or. y?=w205:bool)
    n322 = Or(x=w205, y="Motor stop") -> (x .or. y?=w207:bool)
    n323 = Or(x=w207, y="stop") -> (x .or. y?=w227:bool)
    n324 = Select(t=0.0, s=w227, f=w51) -> (s? t:f=w224:dbl)
    n325 = call-poly <vilib>:"DAQmx Write.vi"("task/channels in"=w233, "data"=w224, "error in"=w230) -> ("task out"=w234:refnum<k21>, "error out"=w235:errorcluster)  [unwired: 10 in, 1 out]
    n326 = Select(t=0.0 ("s? t:f"), s=w227, f=w52) -> (s? t:f=w225:dbl)
    n327 = call-poly <vilib>:"DAQmx Write.vi"("task/channels in"=w239, "data"=w225, "error in"=w229) -> ("task out"=w238:refnum<k21>, "error out"=w237:errorcluster)  [unwired: 10 in, 1 out]
    n328 = call <vilib>:"DAQmx Wait Until Done.vi"("task/channels in"=w238, "error in"=w237) -> ("error out"=w236:errorcluster)  [unwired: 12 in, 1 out]
    n329 = call <vilib>:"DAQmx Wait Until Done.vi"("task/channels in"=w234, "error in"=w235) -> ("error out"=w232:errorcluster)  [unwired: 12 in, 1 out]
    n330 = case shown="True" w128 {
      tunnel: w129 -> [w241 w242]
      frame False {
        n331 = call-poly <vilib>:"DAQmx Read.vi"("task/channels in"=w241) -> ("data"=w240:dbl)  [unwired: 12 in, 2 out]
        n332 = local write "Pulses M2"(w240) -> ()
      }
      frame True {
        n333 = local read "Has encoders been reset?"() -> (w243:enum16{"don't reset", "reset"})
        n334 = case shown="\"reset\"" w243 {
          tunnel: w242 -> [w245 w248]
          frame "don't reset", Default {
            n335 = call-poly <vilib>:"DAQmx Read.vi"("task/channels in"=w245) -> ("data"=→"Pulses M2":dbl)  [unwired: 12 in, 2 out]
          }
          frame "reset" {
            n336 = call <vilib>:"DAQmx Stop Task.vi"("task/channels in"=w248) -> ("task out"=w247:refnum<k21>)  [unwired: 13 in, 1 out]
            n337 = call <vilib>:"DAQmx Start Task.vi"("task/channels in"=w247) -> ("task out"=w249:refnum<k21>)  [unwired: 13 in, 1 out]
            n338 = call-poly <vilib>:"DAQmx Read.vi"("task/channels in"=w249) -> ("data"=w246:dbl)  [unwired: 12 in, 2 out]
            n339 = local write "Pulses M2"(w246) -> ()
          }
        }
      }
    }
    n340 = call "Number To Enum.vim"("number"=w165, "enum type"=enum16{"corner", "1st switch", "reverse"}."corner") -> ("number as enum"=→"Shape drawing steps":enum16{"corner", "1st switch", "reverse"})
    n341 = case shown="True" w128 {
      tunnel: w133 -> [w252 w257]
      tunnel: w132 -> [w253 w256]
      tunnel: [w250 w255] -> w131
      frame False {
        n342 = call-poly <vilib>:"DAQmx Read.vi"("task/channels in"=w252, "error in"=w253) -> ("data"=w251:dbl, "error out"=w250:errorcluster)  [unwired: 11 in, 1 out]
        n343 = local write "Pulses M1"(w251) -> ()
      }
      frame True {
        n344 = case shown="\"reset\"" "Has encoders been reset?" {
          tunnel: w257 -> [w261 w268]
          tunnel: w256 -> [w260 w267]
          tunnel: [w258 w269] -> w255
          frame "don't reset", Default {
            n345 = call-poly <vilib>:"DAQmx Read.vi"("task/channels in"=w261, "error in"=w260) -> ("data"=→"Pulses M1":dbl, "error out"=w258:errorcluster)  [unwired: 11 in, 1 out]
          }
          frame "reset" {
            n346 = call <vilib>:"DAQmx Stop Task.vi"("task/channels in"=w268, "error in"=w267) -> ("task out"=w266:refnum<k21>, "error out"=w265:errorcluster)  [unwired: 12 in]
            n347 = call <vilib>:"DAQmx Start Task.vi"("task/channels in"=w266, "error in"=w265) -> ("task out"=w264:refnum<k21>, "error out"=w263:errorcluster)  [unwired: 12 in]
            n348 = call-poly <vilib>:"DAQmx Read.vi"("task/channels in"=w264, "error in"=w263) -> ("data"=w262:dbl, "error out"=w269:errorcluster)  [unwired: 11 in, 1 out]
            n349 = local write "Pulses M1"(w262) -> ()
          }
        }
      }
    }
  }
  n350 = invoke on="motor 1" class="Slide (strict)" method="Reinit To Default"() -> ()  [unwired: 3 in, 3 out]
  n351 = call <vilib>:"Simple Error Handler.vi"("error source (\" \")"="you messed up" ("error source (\" \")"), "error in (no error)"=w48) -> ()  [unwired: 3 in, 5 out]
  n352 = call <vilib>:"Simple Error Handler.vi"("error source (\" \")"="you messed up" ("error source (\" \")"), "error in (no error)"=w45) -> ()  [unwired: 3 in, 5 out]
  n353 = call <vilib>:"DAQmx Clear Task.vi"("task in"=w27, "error in"=w25) -> ()  [unwired: 13 in, 1 out]
  n354 = call <vilib>:"DAQmx Clear Task.vi"("task in"=w17, "error in"=w14) -> ()  [unwired: 13 in, 1 out]
  n355 = call <vilib>:"DAQmx Clear Task.vi"("task in"=w18, "error in"=w15) -> ("error out"=w12:errorcluster)  [unwired: 13 in]
  n356 = call <vilib>:"DAQmx Clear Task.vi"("task in"=w16, "error in"=w13) -> ()  [unwired: 13 in, 1 out]
  n357 = call <vilib>:"Simple Error Handler.vi"("error in (no error)"=w12) -> ()  [unwired: 4 in, 5 out]
  n358 = call <vilib>:"Simple Error Handler.vi"("error source (\" \")"="you messed up" ("error source (\" \")"), "error in (no error)"=w10) -> ()  [unwired: 3 in, 5 out]
